vi "IMAQ Vision Example folder.vi"() -> (0 "Example Image Path":path)   [LabVIEW 2011]
uses:
  <vilib>/registry/registry.llb/Registry SAM.ctl
  <vilib>/registry/registry.llb/Read Registry Value Simple STR.vi
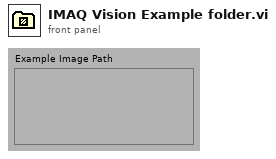
[diagram p1: front panel]
types:
  T1 = typedef "Registry SAM.ctl" = enum32{"KEY_QUERY_VALUE", "KEY_SET_VALUE", "KEY_CREATE_SUB_KEY", "KEY_ENUMERATE_SUB_KEYS", "KEY_NOTIFY", "KEY_CREATE_LINK", "KEY_READ", "KEY_WRITE", "KEY_ALL_ACCESS", "KEY_READ | KEY_WRITE"}
  T2 = typedef "Registry refnum.ctl" = refnum<k1>
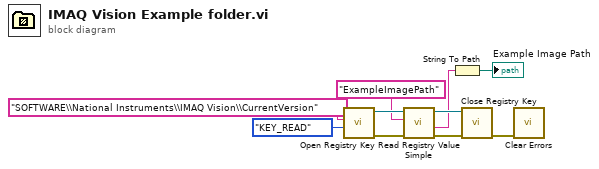
[diagram p0: block diagram]
diagram:
  n1 = call <vilib>:"Open Registry Key.vi"("security access mask (KEY_READ | KEY_WRITE)"=Registry_SAM."KEY_READ", "subkey"="SOFTWARE\\National Instruments\\IMAQ Vision\\CurrentVersion") -> ("error out"=w8:errorcluster, "refnum out"=w7:T2)  [unwired: 2 in, 6 out]
  n2 = call-poly <vilib>:"Read Registry Value Simple.vi"("error in (no error)"=w8, "value"="ExampleImagePath", "refnum"=w7) -> ("error out"=w5:errorcluster, "String/Binary data"=w3:string, "refnum out"=w4:T2)  [unwired: 1 in, 3 out]
  n3 = String To Path(string=w3) -> (path=→"Example Image Path":path)
  n4 = call <vilib>:"Close Registry Key.vi"("error in (no error)"=w5, "refnum"=w4) -> ("error out"=w2:errorcluster)  [unwired: 5 out]
  n5 = call <vilib>:"Clear Errors.vi"("error in (no error)"=w2) -> ()  [unwired: 7 out]
